vi "Write to File.vi"(8 "error in (no error)":errorcluster, 11 "TDMS Report in":refnum<class "Wind TDMS Report.lvclass">) -> (0 "error out":errorcluster, 3 "TDMS Report out":refnum<class "Wind TDMS Report.lvclass">)   [LabVIEW 2009, in "Wind TDMS Report.lvclass"]
doc: "This VI is a dynamic dispatch that overrides the parent method.\n\nAAL 9/09"
uses:
  Wind TDMS Report.lvclass
  Wind Report/Wind Report.lvclass
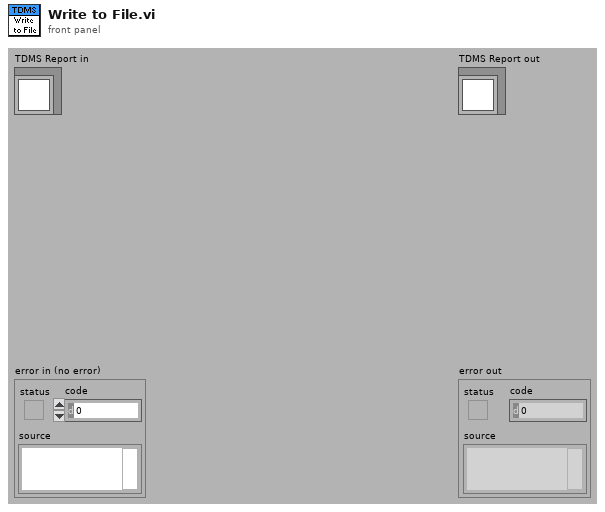
[diagram p1: front panel]
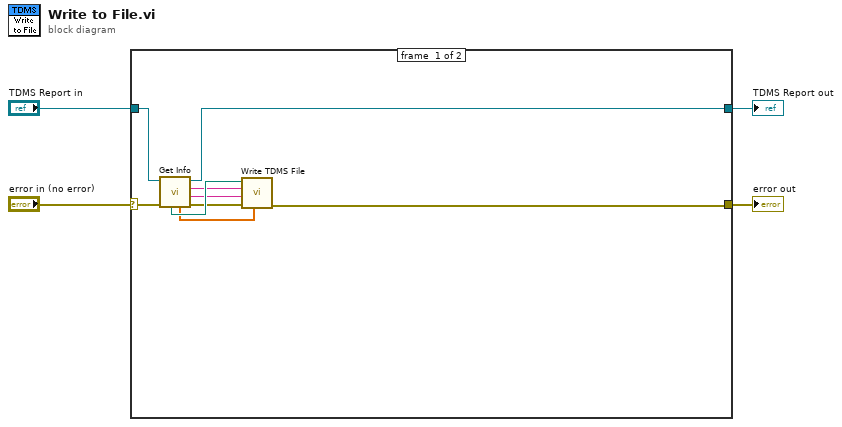
[diagram p0: block diagram]
diagram:
  n1 = case shown="No Error" "error in (no error)" {
    selector: "error in (no error)" -> [w11 w15]
    tunnel: [w8 w15] -> w3
    tunnel: [w12 w14] -> w1
    tunnel: "TDMS Report in" -> [w13 w14]
    frame #0 {
      n2 = call "Get Info.vi"("error in (no error)"=w11, "Report.lvclass in"=w13) -> ("error out"=w9:errorcluster, "Data & Time String"=w6:string, "Header"=w7:string, "Report.lvclass out"=w12:refnum<class "Wind TDMS Report.lvclass">, "Data Array"=w5:dbl[], "Path"=w10:path)  [unwired: 3 in, 1 out]
      n3 = call "Write TDMS File.vi"("Data Array"=w5, "error in"=w9, "Data & Time String"=w6, "Header"=w7, "Path"=w10) -> ("error out"=w8:errorcluster)  [unwired: 6 in]
    }
    frame #1 {
    }
  }
  "error out" <- w3
  "TDMS Report out" <- w1
